vi "chaos crest open.vi"(11 "chaoswanurl":string) -> (3 "connectionHandle":u32)   [LabVIEW 2014, in "libcommon-crest.lvlib"]
doc: "chaos_crest_handle_t chaos_crest_open(const char* chaoswanurl);"
uses:
  libcommon-crest.lvlib
  chaos-i686-dynamic-release/lib/libcommon-crest.so
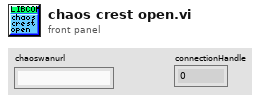
[diagram p1: front panel]
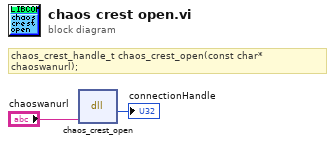
[diagram p0: block diagram]
diagram:
  # "chaos_crest_handle_t chaos_crest_open(const char* chaoswanurl);"
  n1 = dll-call lib="home/chaos/chaos_bundle/chaos-i686-dynamic-release/lib/libcommon-crest.*" fn="chaos_crest_open"("chaoswanurl"="chaoswanurl") -> (→"connectionHandle":u32)  [unwired: 4 in, 2 out]
